vi "reset.vi"(8 "error in (no error)":errorcluster, 11 "DL090623TwoDAnalyser in":refnum<class "AnalyserDL090623TwoD.lvclass">) -> (0 "error out":errorcluster, 3 "DL090623TwoDAnalyser out":refnum<class "AnalyserDL090623TwoD.lvclass">)   [LabVIEW 2010, in "AnalyserDL090623TwoD.lvclass"]
uses:
  AnalyserDL090623TwoD.lvclass
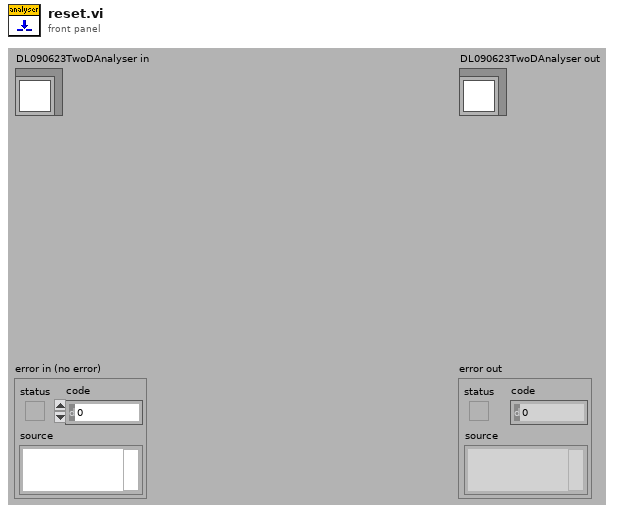
[diagram p1: front panel]
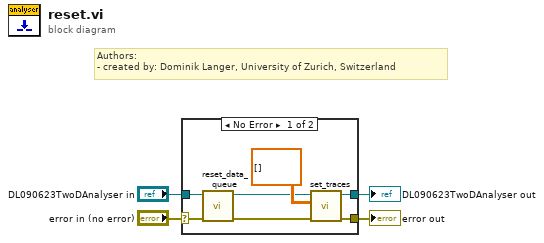
[diagram p0: block diagram]
diagram:
  # "Authors: \n- created by: Dominik Langer, University of Zurich, Switzerland"
  n1 = case shown="No Error" "error in (no error)" {
    selector: "error in (no error)" -> [w8 w13]
    tunnel: [w9 w13] -> w3
    tunnel: [w10 w12] -> w1
    tunnel: "DL090623TwoDAnalyser in" -> [w6 w12]
    frame No Error {
      n2 = call-dynamic "reset_data_queue.vi"("error in (no error)"=w8, "GenericToplevelComponent in"=w6) -> ("error out"=w7:errorcluster, "GenericToplevelComponent out"=w5:refnum<class "AnalyserDL090623TwoD.lvclass">)  [unwired: 8 in]
      n3 = call-dynamic "set_traces.vi"("error in (no error)"=w7, "traces (indices: ROI, sample)"=sgl[][] [], "DL090623TwoDAnalyser.lvclass in"=w5) -> ("error out"=w9:errorcluster, "DL090623TwoDAnalyser.lvclass out"=w10:refnum<class "AnalyserDL090623TwoD.lvclass">)  [unwired: 7 out]
    }
    frame Error {
    }
  }
  "error out" <- w3
  "DL090623TwoDAnalyser out" <- w1
